vi "Power Off.vi"(8 "error in":errorcluster, 11 "Electronic Load in":refnum<class "Electronic Load.lvclass">) -> (0 "error out":errorcluster, 3 "Electronic Load out":refnum<class "Electronic Load.lvclass">)   [LabVIEW 2019, in "Electronic Load.lvlib" / "Electronic Load.lvclass"]
uses:
  Library/Electronic Load.lvclass
  Library/Electronic Load.lvclass/Electronic Load.ctl
  Accessors/Write Active Channel.vi
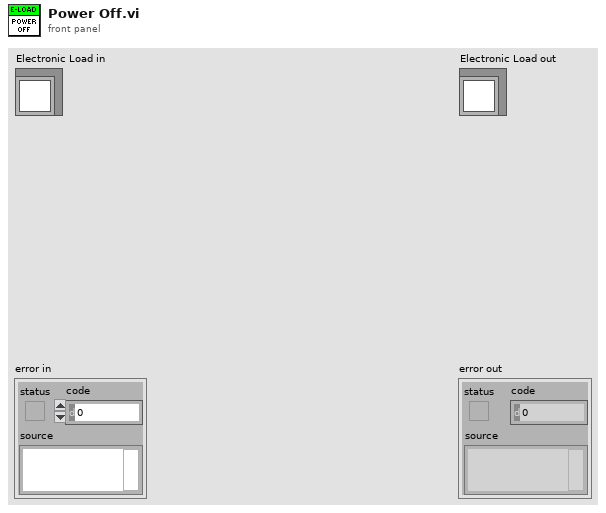
[diagram p1: front panel]
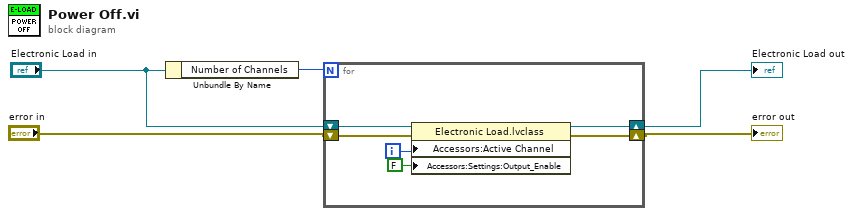
[diagram p0: block diagram]
diagram:
  n1 = Unbundle By Name("Electronic Load in") -> ("Number of Channels"=w5:i32)
  n2 = for {
    N: w5 -> [_]
    shift-right: [w10] -> w3
    shift-left: "Electronic Load in" -> [w11]
    shift-right: [w7] -> w1
    shift-left: "error in" -> [w6]
    i -> [w9]
    n3 = property class="Electronic Load.lvclass"(reference=w11, error in=w6, "Accessors:Active Channel"=w9, "Accessors:Settings:Output_Enable"=FALSE ("Eload:Settings:Output_Enable")) -> (reference out=w10:refnum<class "Electronic Load.lvclass">, error out=w7:errorcluster)
  }
  "error out" <- w1
  "Electronic Load out" <- w3
